vi "Init class.vi"(8 "error in (no error)":errorcluster, 11 "AutoExp in":refnum<class "AutoExp.lvclass">) -> (0 "error out":errorcluster, 3 "AutoExp out":refnum<class "AutoExp.lvclass">)   [LabVIEW 2018, in "AutoExp.lvclass"]
uses:
  AutoExp.lvclass
  Channel/Channel.lvclass
  Channel/Channel.lvclass/Channel.ctl
  AutoExp.lvclass/AutoExp.ctl
panel:
  in  "Channel.lvclass":refnum<class "Channel.lvclass">
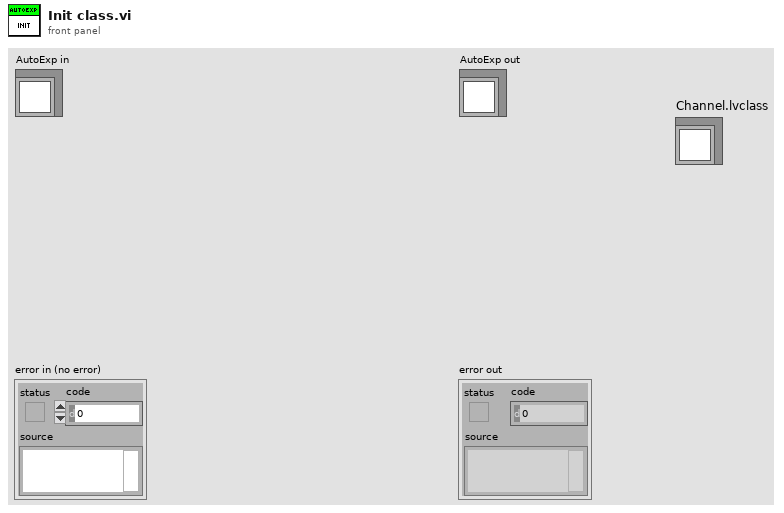
[diagram p1: front panel]
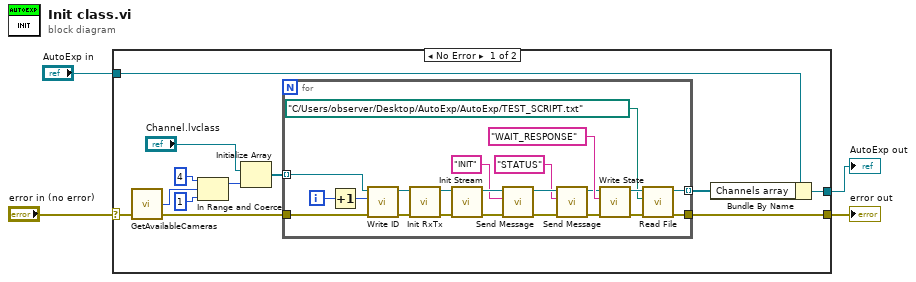
[diagram p0: block diagram]
diagram:
  n1 = case shown="No Error" "error in (no error)" {
    selector: "error in (no error)" -> [w12 w39]
    tunnel: [w7 w40] -> w2
    tunnel: "AutoExp in" -> [w8 w40]
    tunnel: [w5 w39] -> w1
    frame No Error {
      n2 = call <userlib>:"GetAvailableCameras.vi"("error in (no error)"=w12) -> ("error out"=w9:errorcluster, "totalCameras"=w16:i32)  [unwired: 2 in, 1 out]
      n3 = In Range and Coerce(upper limit=4, x=w16, lower limit=1 ("upper limit")) -> (coerced(x)=w13:i32)  [unwired: 1 out]
      n4 = Initialize Array("Channel.lvclass", w13) -> (w10:refnum<class "Channel.lvclass">[])
      n5 = for {
        tunnel: w10 -> [w37] mode=indexing
        tunnel: w9 -> [w38]
        tunnel: [w18] -> w6 mode=indexing
        tunnel: [w19] -> w5
        i -> [w35]
        n6 = Increment(x=w35) -> (x+1=w36:i32)
        n7 = call "Write ID.vi"("error in (no error)"=w38, "ID"=w36, "Channel in"=w37) -> ("error out"=w33:errorcluster, "Channel out"=w34:refnum<class "Channel.lvclass">)  [unwired: 7 in]
        n8 = call "Init RxTx.vi"("error in (no error)"=w33, "Channel in"=w34) -> ("error out"=w31:errorcluster, "Channel out"=w32:refnum<class "Channel.lvclass">)  [unwired: 8 in]
        n9 = call "Init Stream.vi"("error in (no error)"=w31, "Channel in"=w32) -> ("error out"=w29:errorcluster, "Channel out"=w30:refnum<class "Channel.lvclass">)  [unwired: 8 in]
        n10 = call "Send Message.vi"("error in (no error)"=w29, "message"="INIT", "Channel in"=w30) -> ("error out"=w23:errorcluster, "Channel out"=w26:refnum<class "Channel.lvclass">)  [unwired: 7 in]
        n11 = call "Send Message.vi"("error in (no error)"=w23, "message"="STATUS", "Channel in"=w26) -> ("error out"=w24:errorcluster, "Channel out"=w25:refnum<class "Channel.lvclass">)  [unwired: 7 in]
        n12 = call "Write State.vi"("error in (no error)"=w24, "State"="WAIT_RESPONSE" ("message"), "Channel in"=w25) -> ("error out"=w20:errorcluster, "Channel out"=w21:refnum<class "Channel.lvclass">)  [unwired: 7 in]
        n13 = call "Read File.vi"("error in (no error)"=w20, "file path (use dialog)"=path "C:/Users/observer/Desktop/AutoExp/AutoExp/TEST_SCRIPT.txt", "Channel in"=w21) -> ("error out"=w19:errorcluster, "Channel out"=w18:refnum<class "Channel.lvclass">)  [unwired: 7 in]
      }
      n14 = Bundle By Name(cluster=w8, "Channels array"=w6) -> (w7:refnum<class "AutoExp.lvclass">)
    }
    frame Error {
    }
  }
  "error out" <- w1
  "AutoExp out" <- w2
